vi "Wait on Async Calls.vi"(8 "error in (no error)":errorcluster, 10 "Execute VI ref":refnum<vi>) -> (0 "error out":errorcluster, 2 "Suite Results":T1[](array[typedef]))   [LabVIEW 2020, in "Parallell Test Runner.lvclass"]
uses:
  Parallell Test Runner.lvclass
  Core/Runnable/Runnable.lvclass
  Core/Result/Result.ctl
  Core/Result/Status.ctl
  Core/Result/Type.ctl
  Core/Result/Result.lvlib
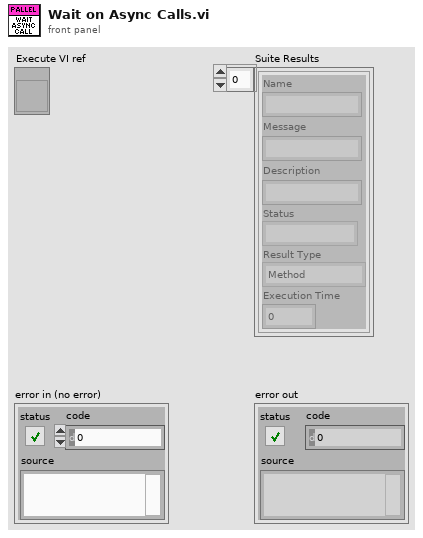
[diagram p1: front panel]
types:
  T1 = typedef "Result.lvlib/Result.ctl" = cluster{"Name":string, "Message":string, "Description":string, "Status":T2, "Result Type":T3, "Execution Time":dbl}
  T2 = typedef "Result.lvlib/Status.ctl" = enum16{"", "Passed", "Failed", "Error", "Skipped", "Setup Error", "Broken", "Teardown Error"}
  T3 = typedef "Result.lvlib/Type.ctl" = enum16{"Method", "Case", "Suite", "Pass", "Fail", "Skip", "Pass if", "Fail if", "Pass if Error", "Fail if Error", "Pass if Equal", "Fail if Equal"}
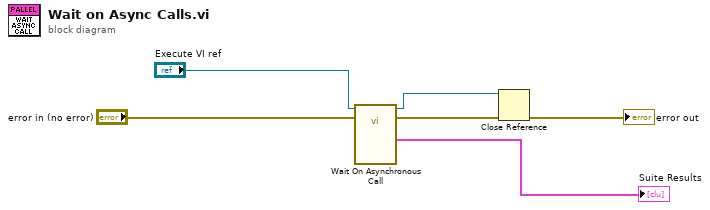
[diagram p0: block diagram]
diagram:
  n1 = call-by-ref "Wait On Asynchronous Call"(reference="Execute VI ref", error in="error in (no error)") -> (reference out=w1:refnum<vi>, error out=w5:errorcluster, "Suite Results"=→"Suite Results":T1[])  [unwired: 11 in]
  n2 = Close Reference(reference=w1, error in (no error)=w5) -> (error out=→"error out":errorcluster)
